vi "Display.vi"(7 "Inverse Mode (F:OFF)":bool, 8 "error in (no error)":errorcluster {"code" format="%.0x"}, 9 "Contrast (0.77)":dbl(knob)=0.768 scale=0.0..10.0 scale format="%.6f", 10 "Brightness (1)":dbl(knob)=1.0 scale=0.0..10.0 scale format="%.1f", 11 "VISA Resource Name":refnum<visa-resource-name>) -> (0 "error out":errorcluster {"code" format="%.0x"}, 3 "VISA Resource Name Out":refnum<visa-resource-name>)   [LabVIEW 2014, in "Agilent ESG Series.lvlib"]
doc: "This VI is used to set the controls and parameters associated with the signal source's LCD display"
uses:
  Agilent ESG Series.lvlib
panel:
  # "ON"
  # "OFF"
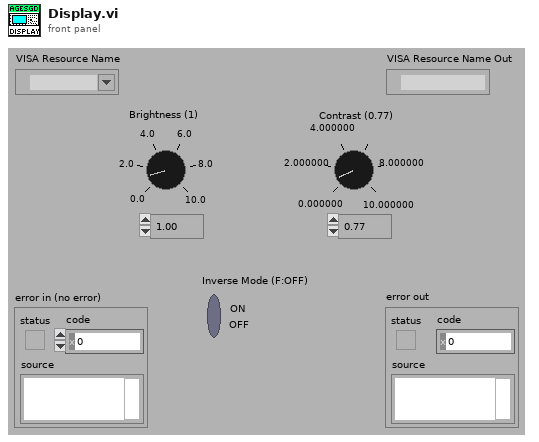
[diagram p1: front panel]
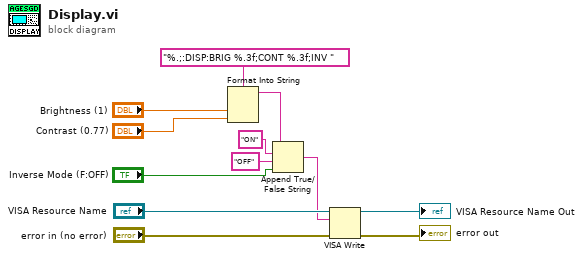
[diagram p0: block diagram]
diagram:
  n1 = Format Into String(format string="%.;:DISP:BRIG %.3f;CONT %.3f;INV ", "Brightness (1)", "Contrast (0.77)") -> (resulting string=w3:string)  [unwired: 2 in, 1 out]
  n2 = Append True/False String(1:"Inverse Mode (F:OFF)", 2:"OFF" ("false string"), 3:"ON" ("true string"), 4:w3) -> (0:w1:string)
  n3 = VISA Write(VISA resource name="VISA Resource Name", write buffer=w1, error in (no error)="error in (no error)") -> (VISA resource name out=→"VISA Resource Name Out":refnum<visa-resource-name>, error out=→"error out":errorcluster)  [unwired: 1 out]
